vi "ReadGroupedDigitalOutputs.vi"(8 "error in (no error)":errorcluster, 11 "DigitalOutput_Simulation In":refnum<class "TesteractHAL_DigitalOutput_Simulation.lvclass">) -> (0 "error out":errorcluster, 2 "data":u32, 3 "DigitalOutput_Simulation Out":refnum<class "TesteractHAL_DigitalOutput_Simulation.lvclass">)   [LabVIEW 2017, in "TesteractHAL_DigitalOutput_Simulation.lvlib" / "TesteractHAL_DigitalOutput_Simulation.lvclass"]
doc: "Read 1 sample of a single channel containing multiple digital signals."
uses:
  TesteractHAL_DigitalOutput_Simulation.lvclass
  TesteractHAL_DigitalOutput_Simulation.lvclass/TesteractHAL_DigitalOutput_Simulation.ctl
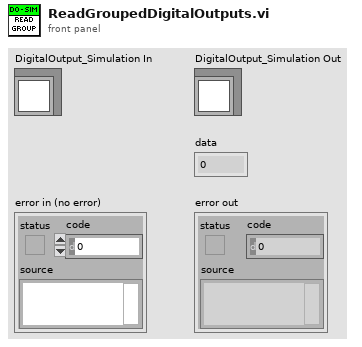
[diagram p1: front panel]
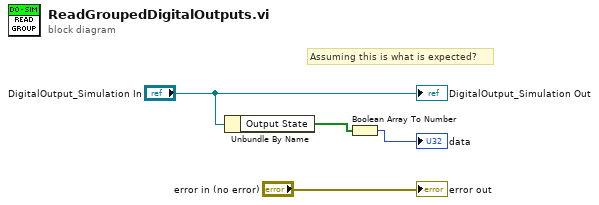
[diagram p0: block diagram]
diagram:
  # "Assuming this is what is expected?"
  n1 = Unbundle By Name("DigitalOutput_Simulation In") -> ("Output State"=w2:bool[])
  n2 = Boolean Array To Number(Boolean array=w2) -> (number=→"data":u32)
  "error out" <- "error in (no error)"
  "DigitalOutput_Simulation Out" <- "DigitalOutput_Simulation In"
